vi "Lookup Command Info.vi"(8 "error in (no error)":errorcluster, 10 "Channel Lookup Info in":T6 {"Refs" format="%.0x"}, 11 "Item Ref in":T3 format="%.0x") -> (0 "error out":errorcluster, 1 "Command Parameters":T4, 2 "Channel Lookup Info out":T6 {"Refs" format="%.0x"}, 3 "Section Ref out":T3 format="%.0x", 5 "Command Channel Indeces":T1)   [LabVIEW 2019, in "Instrument Addon System Explorer.lvlib"]
uses:
  Instrument Addon System Explorer.lvlib
  Types/Channel Lookup Cluster.ctl
  <vilib>/NI VeriStand/Custom Device API/Custom Device Item Ref.ctl
  Addon Shared/Types/Command Parameters.ctl
  Addon Shared/Types/Linked Channel Cluster.ctl
  Addon Shared/Types/Command Channel Indeces.ctl
  Addon Shared/Types/Command Channel Index.ctl
  Addon Shared/Types/FG Control.ctl
  Addon Shared/Types/Meta Data RT Configuration Cluster.ctl
  Addon Shared/Types/MetaData Parameters.ctl
  Addon Shared/Types/Protocol Data Type.ctl
  Addon Shared/Types/Metadata Channel Type.ctl
  Addon Shared/Types/Type Cast Type.ctl
  Addon Shared/Types/Endian.ctl
  Addon Shared/SubVIs/MetaData Parameters FG.vi
  Addon Shared/SubVIs/Constants.vi
  <vilib>/NI VeriStand/Custom Device Tools/Custom Device Utility Library/NI VeriStand - Search for Item by GUID.vi
  <vilib>/NI VeriStand/Custom Device API/NI VeriStand - Get Item Property.vi
  <vilib>/NI VeriStand/Custom Device API/Get Item Property (String).vi
  <vilib>/NI VeriStand/Custom Device API/Get Item Property (String Array).vi
  <vilib>/NI VeriStand/Custom Device API/Get Item Property (Boolean).vi
  <vilib>/NI VeriStand/Custom Device API/Get Item Property (U32).vi
  <vilib>/NI VeriStand/Custom Device API/NI VeriStand - Set Item Property.vi
  <vilib>/NI VeriStand/Custom Device API/Set Item Property (String).vi
  <vilib>/NI VeriStand/Custom Device API/Set Item Property (String Array).vi
  <vilib>/NI VeriStand/Custom Device API/Set Item Property (Boolean).vi
  <vilib>/NI VeriStand/Custom Device API/Set Item Property (U32).vi
  Addon Shared/SubVIs/Set Channel Value Table.vi
  <vilib>/NI VeriStand/Custom Device Tools/Custom Device Utility Library/Custom Device Utility Library.lvlib
  Addon Shared/Instrument Addon Shared.lvlib
  <vilib>/NI VeriStand/Custom Device API/Custom Device API.lvlib
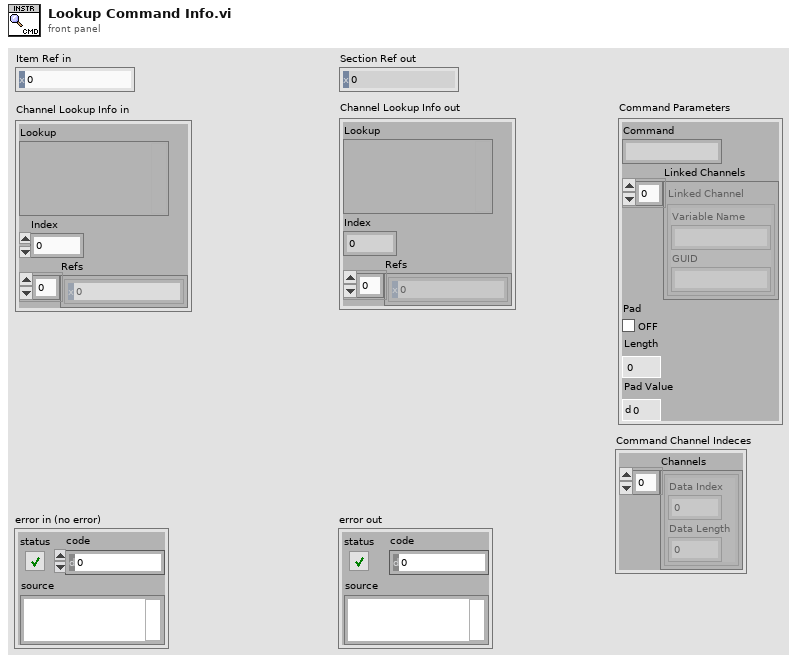
[diagram p1: front panel]
types:
  T1 = typedef "Instrument Addon Shared.lvlib/Command Channel Indeces.ctl" = cluster{"Channels":T2[]}
  T2 = typedef "Instrument Addon Shared.lvlib/Command Channel Index.ctl" = cluster{"Data Index":i32, "Data Length":i32}
  T3 = typedef "Custom Device API.lvlib/Custom Device Item Ref.ctl" = u64
  T4 = typedef "Instrument Addon Shared.lvlib/Command Parameters.ctl" = cluster{"Command":string, "Linked Channels":T5[], "Pad":bool, "Length":u32, "Pad Value":u8}
  T5 = typedef "Instrument Addon Shared.lvlib/Linked Channel Cluster.ctl" = cluster{"Variable Name":string, "GUID":string}
  T6 = typedef "Instrument Addon System Explorer.lvlib/Channel Lookup Cluster.ctl" = cluster{"Lookup":variant, "Index":i32, "Refs":T3[]}
  T7 = typedef "Instrument Addon Shared.lvlib/FG Control.ctl" = enum16{"Get", "Set"}
  T8 = typedef "Instrument Addon Shared.lvlib/Meta Data RT Configuration Cluster.ctl" = cluster{"MetaData Parameters":T9, "Data Index":i32, "Data Length":i32}
  T9 = typedef "Instrument Addon Shared.lvlib/MetaData Parameters.ctl" = cluster{"Data Type":T10, "Channel Type":T11, "List":string[], "Format String":string, "Type":T12, "Delimiter":string, "Endian":T13}
  T10 = typedef "Instrument Addon Shared.lvlib/Protocol Data Type.ctl" = enum16{"Single Channel", "Array"}
  T11 = typedef "Instrument Addon Shared.lvlib/Metadata Channel Type.ctl" = enum16{"Enumerated List", "Format", "Type Cast"}
  T12 = typedef "Instrument Addon Shared.lvlib/Type Cast Type.ctl" = enum16{"DBL", "SGL", "U64", "U32", "U16", "U8", "I64", "I32", "I16", "I8"}
  T13 = typedef "Instrument Addon Shared.lvlib/Endian.ctl" = enum16{"Native", "Little", "Big"}
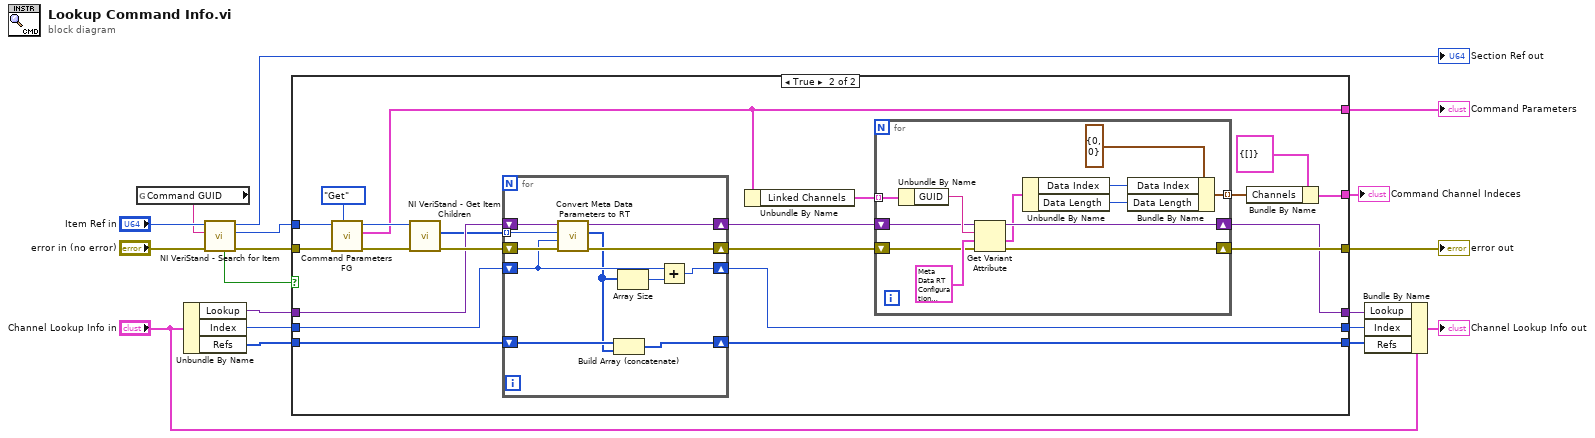
[diagram p0: block diagram]
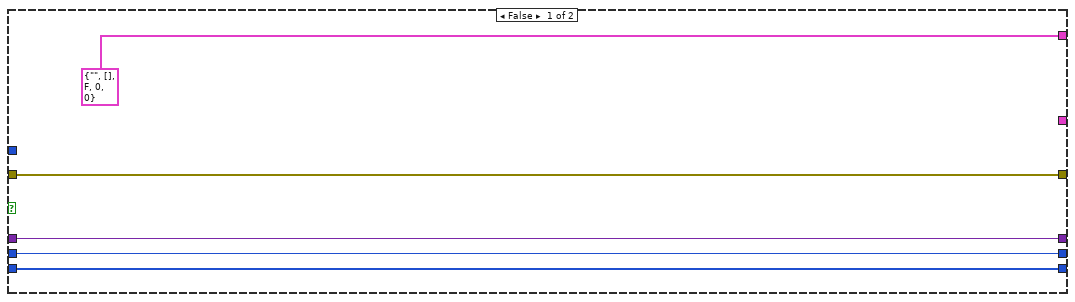
[diagram p2: hidden frame]
diagram:
  n1 = global read "Constants.vi" "Command GUID"() -> (w2:string)
  n2 = Unbundle By Name("Channel Lookup Info in") -> ("Lookup"=w11:variant, "Index"=w12:i32, "Refs"=w13:T3[])
  n3 = call-poly <vilib>:"NI VeriStand - Search for Item.vi"("error in"="error in (no error)", "Item GUID"=w2, "Section Ref in"="Item Ref in") -> ("error out"=w3:errorcluster, "Item Ref"=w5:T3, "Section Ref out"=→"Section Ref out":T3, "Found"=w8:bool)  [unwired: 5 in]
  n4 = case shown="True" w8 {
    tunnel: w3 -> [w23 w44]
    tunnel: [w23 w29] -> w4
    tunnel: w11 -> [w22 w39]
    tunnel: [w20 w33] -> w17
    tunnel: w13 -> [w20 w34]
    tunnel: w12 -> [w21 w37]
    tunnel: [w21 w36] -> w16
    tunnel: [w22 w27] -> w15
    tunnel: w5 -> [_ w35]
    tunnel: [T4 {"Command"="", "Linked Channels"=[], "Pad"=FALSE, "Length"=0, "Pad Value"=0} ("Command Parameters") w32] -> w7
    tunnel: [_ w25] -> w1
    frame False {
    }
    frame True {
      n5 = call "Command Parameters FG.vi"("Action"=FG_Control."Get", "error in (no error)"=w44, "Item Ref in"=w35) -> ("error out"=w42:errorcluster, "Command Parameters"=w32:T4, "Item Ref out"=w40:T3)  [unwired: 6 in]
      n6 = call <vilib>:"NI VeriStand - Get Item Children.vi"("error in (no error)"=w42, "Item Ref in"=w40) -> ("error out"=w41:errorcluster, "Child Refs"=w38:T3[])  [unwired: 6 in, 2 out]
      n7 = for {
        shift-right: [w62] -> w30
        shift-left: w41 -> [w66]
        tunnel: w38 -> [w65] mode=indexing
        shift-right: [w67] -> w36
        shift-left: w37 -> [w60]
        shift-right: [w63] -> w28
        shift-left: w39 -> [w64]
        shift-right: [w58] -> w33
        shift-left: w34 -> [w59]
        n8 = call "Convert Meta Data Parameters to RT.vi"("error in (no error)"=w66, "Data Index"=w60, "Item Ref in"=w65, "Lookup Table"=w64) -> ("error out"=w62:errorcluster, "Chan Refs"=w57:T3[], "Lookup Table out"=w63:variant)  [unwired: 5 in]
        n9 = Build Array (concatenate)(w59, w57) -> (w58:T3[])
        n10 = Array Size(array=w57) -> (size(s)=w61:i32)
        n11 = Add(x=w60, y=w61) -> (x+y=w67:i32)
      }
      n12 = Unbundle By Name(w32) -> ("Linked Channels"=w31:T5[])
      n13 = for {
        tunnel: w31 -> [w55] mode=indexing
        shift-right: [w52] -> w29
        shift-left: w30 -> [w53]
        shift-right: [w50] -> w27
        shift-left: w28 -> [w51]
        tunnel: [w46] -> w26 mode=indexing
        n14 = Unbundle By Name(w55) -> ("GUID"=w54:string)
        n15 = Get Variant Attribute(Variant=w51, name=w54, default value (empty Variant)=T8 {"MetaData Parameters"={"Data Type"=enum."Single Channel", "Channel Type"=enum."Enumerated List", "List"=[], "Format String"="", "Type"=enum."DBL", "Delimiter"="", "Endian"=enum."Native"}, "Data Index"=0, "Data Length"=0}, error in=w53) -> (duplicate Variant=w50:variant, value=w49:T8, error out=w52:errorcluster)  [unwired: 1 out]
        n16 = Unbundle By Name(w49) -> ("Data Index"=w48:i32, "Data Length"=w47:i32)
        n17 = Bundle By Name(cluster=T2 {"Data Index"=0, "Data Length"=0}, "Data Index"=w48, "Data Length"=w47) -> (w46:T2)
      }
      n18 = Bundle By Name(cluster=T1 {"Channels"=[]} ("Command Channel Indeces"), "Channels"=w26) -> (w25:T1)
    }
  }
  "Command Parameters" <- w7
  "error out" <- w4
  "Command Channel Indeces" <- w1
  n19 = Bundle By Name(cluster="Channel Lookup Info in", "Lookup"=w15, "Index"=w16, "Refs"=w17) -> (→"Channel Lookup Info out":T6)
